vi "Load Categories.vi"(8 "error in (no error)":errorcluster, 11 "Budgetizer in":refnum<class "Budgetizer.lvclass">) -> (0 "error out":errorcluster, 2 "Names Loaded":string[](array[string]), 3 "Budgetizer out":refnum<class "Budgetizer.lvclass">)   [LabVIEW 2018, in "Budgetizer.lvclass"]
uses:
  Budgetizer.lvclass
  Budgetizer.lvclass/Budgetizer.ctl
  database/Database.lvclass
  Category/Category.lvclass
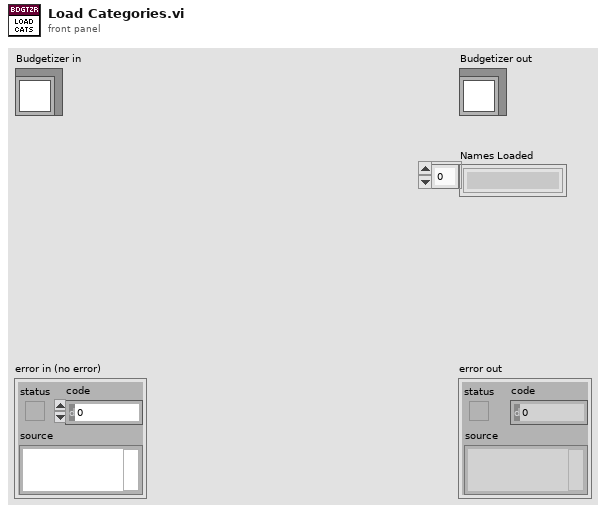
[diagram p1: front panel]
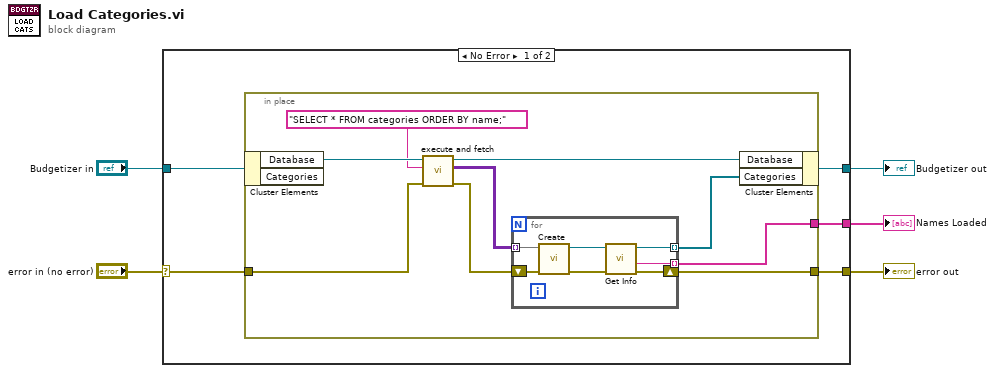
[diagram p0: block diagram]
diagram:
  n1 = case shown="No Error" "error in (no error)" {
    selector: "error in (no error)" -> [w7 w28]
    tunnel: [w8 w28] -> w4
    tunnel: [w9 w27] -> w2
    tunnel: "Budgetizer in" -> [w10 w27]
    tunnel: [w6 _] -> w1
    frame No Error {
      n2 = in-place {
        in-place-border: w7 -> [w17]
        in-place-border: [w13] -> w8
        in-place-border: [w11] -> w6
        n3 = in-place-cluster #1(w10) -> ("Database"=w19:refnum<class "Database.lvclass">)  [unwired: 1 out]
        n4 = call "execute and fetch.vi"("error in (no error)"=w17, "SQL query"="SELECT * FROM categories ORDER BY name;", "Database in"=w19) -> ("error out"=w14:errorcluster, "recordset data"=w15:variant[][], "Database out"=w18:refnum<class "Database.lvclass">)  [unwired: 5 in, 1 out]
        n5 = for {
          tunnel: w15 -> [w26] mode=indexing
          shift-right: [w21] -> w13
          shift-left: w14 -> [w25]
          tunnel: [w22] -> w12 mode=indexing
          tunnel: [w20] -> w11 mode=indexing
          n6 = call "Create.vi"("error in (no error)"=w25, "Record"=w26) -> ("error out"=w23:errorcluster, "Category out"=w24:refnum<class "Category.lvclass">)  [unwired: 8 in]
          n7 = call "Get Info.vi"("error in (no error)"=w23, "Category in"=w24) -> ("error out"=w21:errorcluster, "Name"=w20:string, "Category out"=w22:refnum<class "Category.lvclass">)  [unwired: 6 in, 1 out]
        }
        n8 = in-place-cluster #1("Database"=w18, "Categories"=w12) -> (w9:refnum<class "Budgetizer.lvclass">)
      }
    }
    frame Error {
    }
  }
  "error out" <- w4
  "Budgetizer out" <- w2
  "Names Loaded" <- w1
